vi "Get Filepath.vi"(8 "error in":errorcluster, 11 "FileHandler in":refnum<class "FileHandler.lvclass">) -> (0 "error out":errorcluster, 2 "Filepath":path, 3 "FileHandler out":refnum<class "FileHandler.lvclass">)   [LabVIEW 2020, in "hse-logger.lvlib" / "FileHandler.lvclass"]
doc: "____\nHAMPEL SOFTWARE ENGINEERING v2.0.6 (2021-04-15 11:38)"
uses:
  FileHandler.lvclass
  FileHandler.lvclass/FileHandler.ctl
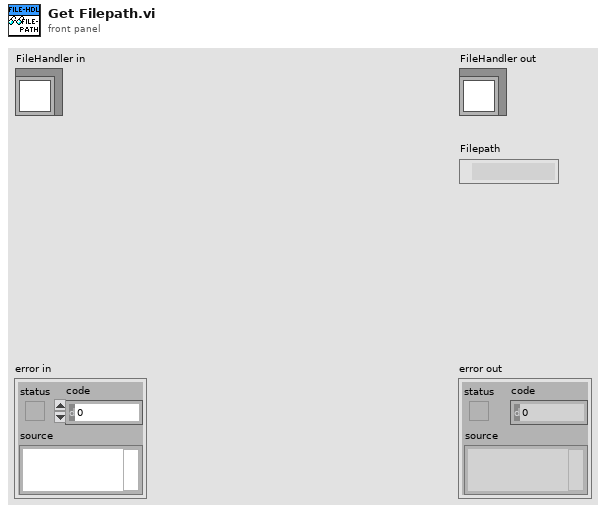
[diagram p1: front panel]
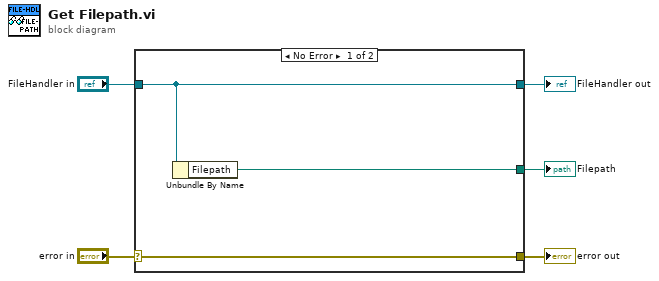
[diagram p0: block diagram]
diagram:
  n1 = case shown="No Error" "error in" {
    selector: "error in" -> [w8 w9]
    tunnel: [w8 w9] -> w4
    tunnel: [w7 w10] -> w2
    tunnel: "FileHandler in" -> [w7 w10]
    tunnel: [w6 _] -> w1
    frame No Error {
      n2 = Unbundle By Name(w7) -> ("Filepath"=w6:path)
    }
    frame Error {
    }
  }
  "error out" <- w4
  "FileHandler out" <- w2
  "Filepath" <- w1
